vi "Vision Processing.vi"(4 "error in (no error)":errorcluster, 7 "Image Size Gear":T6=enum."160x120") -> ()   [LabVIEW 2016]
doc: "This VI runs in parallel to other tasks. It gets images from the camera, processes them for color or shape and use that information to affect robot behavior."
uses:
  Vision Support VIs/Camera Types.ctl
  <vilib>/Rock Robotics/WPI/Camera/WPI_CameraImageSize.ctl
  <vilib>/vision/Measure.llb/Edge Options.ctl
  <vilib>/vision/Measure.llb/Edge Polarity.ctl
  <vilib>/Rock Robotics/WPI/Camera/WPI_CameraWhite Balance Values.ctl
  <vilib>/Rock Robotics/WPI/Camera/WPI_CameraExposure Values.ctl
  <vilib>/Rock Robotics/WPI/Camera/WPI_CameraFrameRate.ctl
  <vilib>/Platform/TimedLoop/XDataNode/timing_clust.ctl
  <vilib>/Platform/TimedLoop/XDataNode/nitl_modes.ctl
  <vilib>/Platform/TimedLoop/XDataNode/wakeup.ctl
  <userlib>/836-libraries/Drive/Drive_Code/Drive_Code_Support/Sensor_Cluster.ctl
  <userlib>/836-libraries/Drive/Drive_Code/Drive_Code_Support/Camera_Cluster.ctl
  <userlib>/836-libraries/Drive/Drive_Code/Drive_Code_Support/Drive_Code_Notifier.ctl
  <userlib>/836-libraries/Drive/Drive_Code/Drive_Code_Support/Drive_Code_Command.ctl
  <userlib>/836-libraries/Drive/Drive_Code/Logging_Data.ctl
  <userlib>/836-libraries/Drive/Drive_Code/Drive_Code_Support/Drive_Code_PID_Bundle.ctl
  <vilib>/Rock Robotics/Network Tables/NT Write Boolean.vi
  <vilib>/platform/TimedLoop/XDataNode/XDataNode.xnode
  <vilib>/vision/NI_Vision_Development_Module.lvlib
  <vilib>/Platform/TimedLoop/XDataNode/XDNodeRunTimeDep.lvlib
panel:
  out "Mode 2":bool
  out "OOR 2":bool=TRUE
  out "GEAR cam":T1(graph)={"Distance (lateral)"=181.92766755741692, "Filtered"=0.0}
  in  "Rate Thresh 2":dbl=30.0 step=0.001
  in  "hi limit 2":dbl=100.0
  out "Distance (CT)":dbl=181.92766755741692
  in  "GearValid":dbl=40.0 format="%#_13g"
  in  "Gear Align % Y":dbl=70.0
  in  "Gear Align Offset (in)":dbl=30.0
  in  "Gear Tgt Sep":dbl=8.0
  in  "Gear Camera Orientation":cluster{"Yaw":dbl, "Elevation":dbl}={"Yaw"=0.0, "Elevation"=-2.0}
  out "Distance (lateral) 2":dbl=237.25608944267697
  out "Distance (lateral) 1":dbl=147.49292175195765
  in  "Hyster":dbl=0.3
  out "Mode":bool=TRUE
  out "OOR":bool
  in  "Rate Thresh":dbl=20.0 step=0.001
  in  "hi limit":dbl=50.0
  out "Waveform Chart":T2(graph)={"Distance (ft)"=inf, "Distance (ft)"=10.013263699521787, "Filtered"=10.013263699521787, "Double"=10.013263699521787}
  in  "Angle 2":enum16{"Horizontal", "Vertical", "Diagonal"}(ring)=enum."Vertical"
  out "Gear Yaw Delta":dbl=-2.9065025252525256
  in  "Boiler boresight":dbl=1.4
  in  "Edge Options Gear":T3={"Edge Polarity"=0, "Kernel Size"=3, "Width"=3, "Minimum Edge Strength"=15.0, "Interpolation Type"=enum."Bilinear Fixed", "Data Processing Method"=enum."Average"} {"Edge Polarity" items=["All Edges", "Rising Edges", "Falling Edges"]; "Minimum Edge Strength" format="%.2f"; "Width" step=2; "Kernel Size" step=2}
  in  "Gear boresight":dbl=-0.8
  in  "Ball?":bool=TRUE
  in  "LED Color Ball":T5={"Hue"={177.87863998678503, 241.41851407789423}, "Sat"={54.64285714285715, 255.0}, "Val"={37.39285714285715, 233.75}} {"Hue" scale=0.0..255.0 scale format="%#_3g"}
  in  "Brightness":i32=30
  in  "Exposure (%)":dbl format="%#_13g"
  in  "Color Temp (K)":dbl=4000.0 format="%#_13g"
  in  "Edge Options":T3={"Edge Polarity"=0, "Kernel Size"=3, "Width"=3, "Minimum Edge Strength"=20.0, "Interpolation Type"=enum."Bilinear Fixed", "Data Processing Method"=enum."Average"} {"Edge Polarity" items=["All Edges", "Rising Edges", "Falling Edges"]; "Minimum Edge Strength" format="%.2f"; "Width" step=2; "Kernel Size" step=2}
  in  "Size Limit %":dbl=0.04 format="%#_13g"
  in  "Cal Turret":bool
  out "Calibration error 2":errorcluster={"status"=TRUE, "code"=-1074396074, "source"=""}
  out "Physical Paths":string[](array[string])=["-0_1_1_1_0", "-0_1_2_1_0"]
  out "Logical Paths":string[](array[string])=["video0", "video1"]
  out "Gear Valid":bool
  out "Boiler Yaw Delta":dbl=-28.4328125
  out "Boiler Valid":bool
  out "Boiler Distance":dbl=inf
  in  "Angle":enum16{"Horizontal", "Vertical", "Diagonal"}(ring)=enum."Vertical"
  in  "Gear?":bool
  in  "Image SizeTurr":T6=enum."160x120"
  in  "Score Cutoff Turret":dbl=70.0
  in  "FOV":cluster{"X (degrees)":dbl, "Y (degrees)":dbl}={"X (degrees)"=61.0, "Y (degrees)"=34.3}
  in  "Height":T7={"Hc (GND to lense)"=4.25, "Ht (GND to CTR)"=13.25}
  in  "LED Color Target":T5={"Hue"={161.40152626725316, 238.59547054989036}, "Sat"={51.60714285714287, 255.0}, "Val"={18.071428571428584, 255.0}} {"Hue" scale=0.0..255.0 scale format="%#_3g"}
  in  "Camera Type":T8=enum."1013"
  in  "Score Cutoff %":dbl=50.0
  in  "Particles":dbl=5.0
  in  "Color Mode":u16(ring)=3 items=["RGB", "HSL", "HSV", "HSI"]
  in  "Use Calibration":bool
  out "Calibration error":errorcluster
  in  "Line Border":cluster{"Top":dbl, "Bottom":dbl}={"Top"=6.0, "Bottom"=1.0}
  in  "Display Original":bool=TRUE
  in  "Display Mask":bool=TRUE
  out "Mask":T9(plugin-control)
  out "Original Image":T9(plugin-control)
  out "loop ms":u32=100
  # "GEAR"
  # "TURRET"
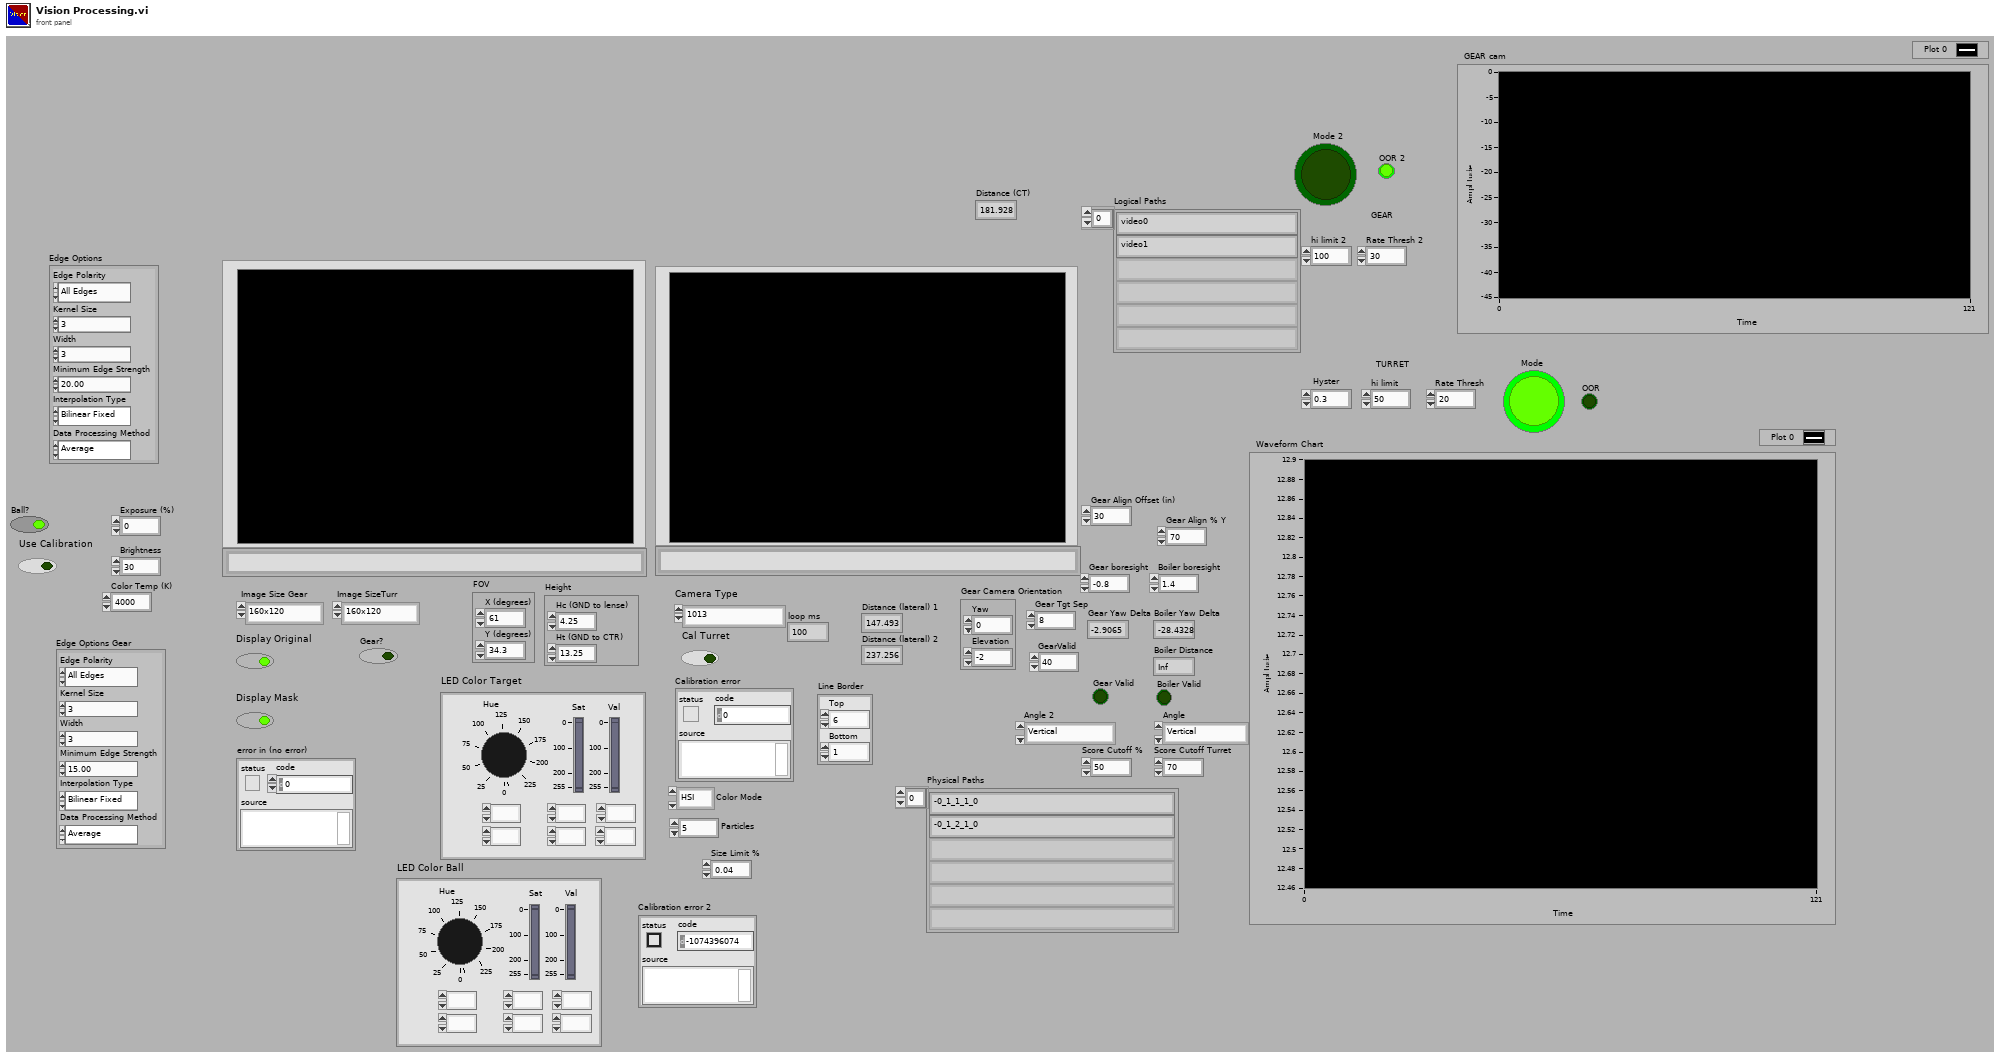
[diagram p1: front panel]
types:
  T1 = cluster{"Distance (lateral)":dbl, "Filtered":dbl}
  T2 = cluster{"Distance (ft)":dbl, "Distance (ft)":dbl, "Filtered":dbl, "Double":dbl}
  T3 = typedef "Edge Options.ctl" = cluster{"Edge Polarity":T4, "Kernel Size":u32, "Width":u32, "Minimum Edge Strength":sgl, "Interpolation Type":enum32{"Zero Order", "Bilinear", "Quadratic", "Cubic", "Bilinear Fixed"}, "Data Processing Method":enum32{"Average", "Median"}}
  T4 = typedef "Edge Polarity.ctl" = u32
  T5 = cluster{"Hue":cluster{dbl, dbl}, "Sat":cluster{dbl, dbl}, "Val":cluster{dbl, dbl}}
  T6 = typedef "WPI_CameraImageSize.ctl" = enum16{"640x480", "320x240", "160x120", "Custom"}
  T7 = cluster{"Hc (GND to lense)":dbl, "Ht (GND to CTR)":dbl}
  T8 = typedef "Camera Types.ctl" = enum16{"206", "1011", "1013", "MS HD3000 square", "MS HD3000 640x480"}
  T9 = typedef "IMAQ Image.ctl" = refnum<image>
  T10 = typedef "Image Type" = u32
  T11 = typedef "WPI_CameraFrameRate.ctl" = u32
  T12 = typedef "WPI_CameraExposure Values.ctl" = enum16{"Auto", "Flicker-free 50 Hz", "Flicker-free 60 Hz", "Hold current", "Custom"}
  T13 = typedef "WPI_CameraWhite Balance Values.ctl" = enum16{"Auto", "Fixed indoor", "Fixed outdoor 1", "Fixed outdoor 2", "Fixed fluorescent 1", "Fixed fluorescent 2", "Hold current", "Custom"}
  T14 = typedef "Particle Parameters" = i32
  T15 = typedef "WPI_CameraDevRef.ctl" = cluster{"Camera Address":string, "CameraStatus":errorcluster}
  T16 = typedef "XDNodeRunTimeDep.lvlib/timing_clust.ctl" = cluster{"Expected End [f-1]":u64, "Actual End [f-1]":u64, "Finished Late? [f-1]":bool, "Expected End [i-1]":u64, "Actual End [i-1]":u64, "Finished Late? [i-1]":bool, "Expected Start [i]":u64, "Actual Start [i]":u64, "Expected Start [f]":u64, "Actual Start [f]":u64, "Source Name":string, "Structure Name":string, "Period":i64, "Deadline":i64, "Offset":i64, "Start":i64, "Priority":i32, "Timeout":i32, "Mode":T17, "Wakeup Reason":T18, "Error":errorcluster, "Source Type":string, "Secondary Source Type":string, "Global End Time":u64, "Global Start Time":u64, "Frame Duration":u64, "Iteration Duration":u64, "Assigned CPU":i32, "I/O Scan Engine Mode":u32}
  T17 = typedef "XDNodeRunTimeDep.lvlib/nitl_modes.ctl" = enum32{"No Change", "Process missed periods, maintain original phase", "Discard missed periods, maintain original phase", "Process missed periods, ignore original phase", "Discard missed periods, ignore original phase"}
  T18 = typedef "XDNodeRunTimeDep.lvlib/wakeup.ctl" = enum32{"Normal", "Aborted", "Asynchronous wakeup", "Timing source error", "Timed loop error", "Timeout"}
  T19 = typedef "Sensor_Cluster.ctl" = cluster{"Gyro Data":cluster{"Gyro RT FIFO":refnum<k33>, "Gyro Current":dbl, "Gyro Hold":dbl}, "Encoder Data":cluster{"Encoder RT FIFO":refnum<k33>, "Encoder Current":dbl, "Encoder Hold":dbl}, "Camera Data":cluster{"Camera RT FIFO":refnum<k33>, "Camera Current":T20}}
  T20 = typedef "Camera_Cluster.ctl" = cluster{" Angle":dbl, "Valid":bool}
  T21 = cluster{"Cluster":T19, "Drive Command rt fifo":refnum<k33>, "Logging Data":refnum<k33>, "PID Update":refnum<notifier>}
  T22 = cluster{"Left":dbl, "Top":dbl, "Right":dbl, "Bottom":dbl}
  T23 = cluster{"Distance (ft)":dbl, "Score":dbl, "Normalized":cluster{"Center":cluster{dbl, dbl}, "Rectangle":cluster{"Numeric":dbl, "Numeric 2":dbl, "Numeric 3":dbl, "Numeric 5":dbl}}, "Pixels":cluster{"Center":cluster{dbl, dbl}, "Rectangle":cluster{"Numeric":dbl, "Numeric 2":dbl, "Numeric 3":dbl, "Numeric 5":dbl}}}
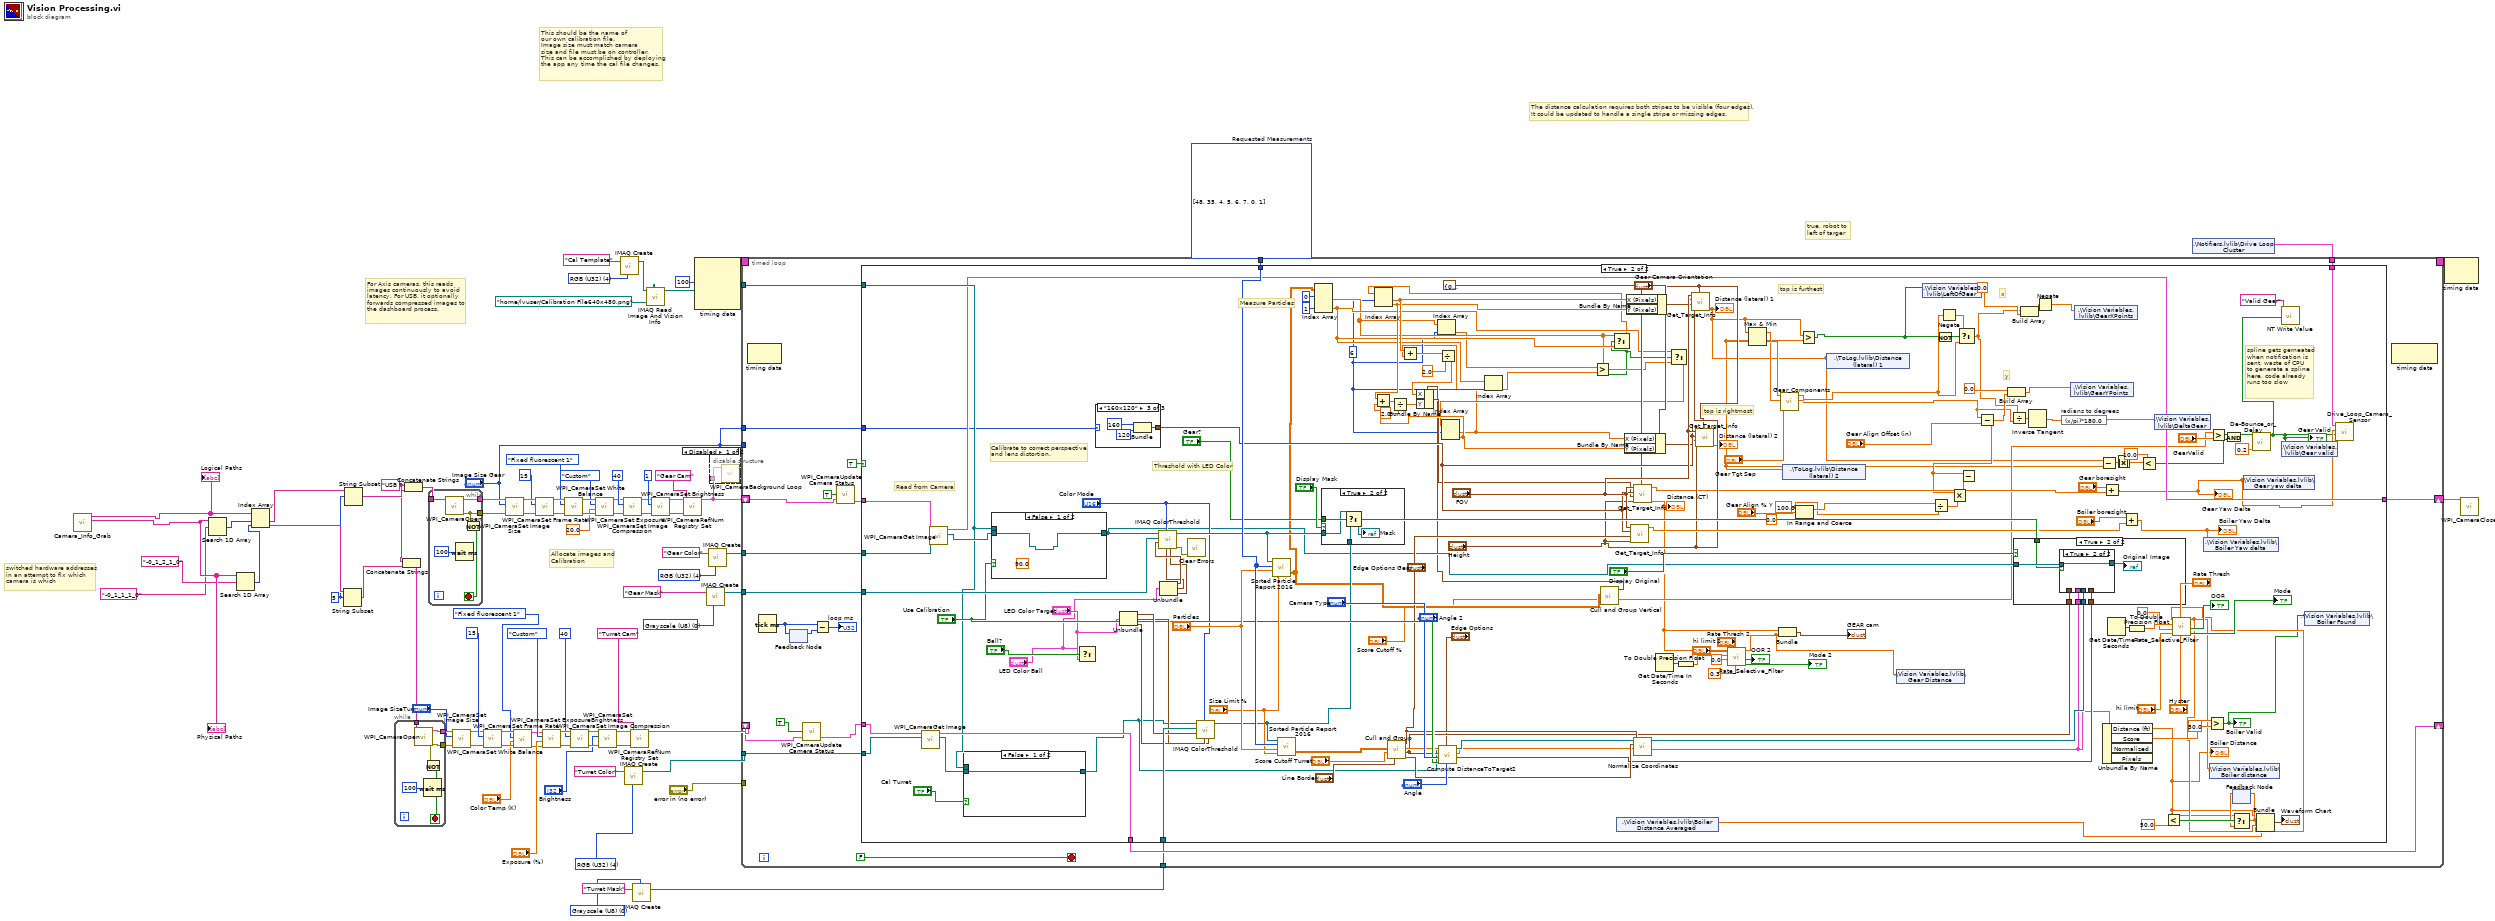
[diagram p0: block diagram]
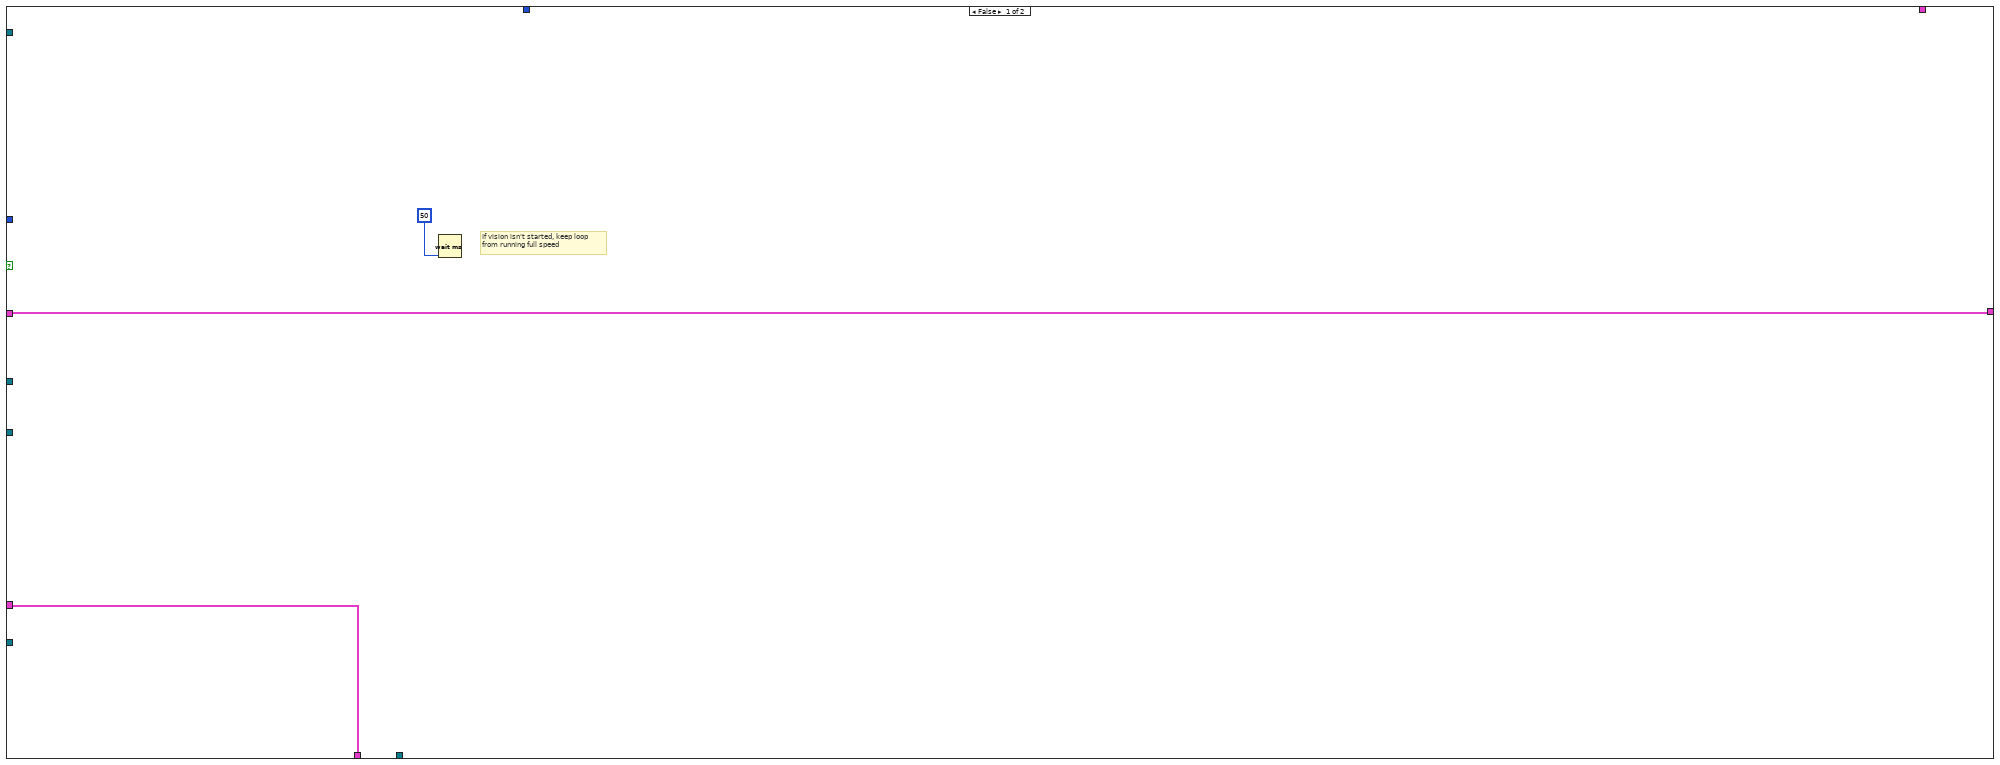
[diagram p2: hidden frame]
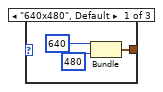
[diagram p3: hidden frame]
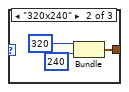
[diagram p4: hidden frame]
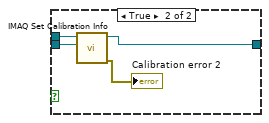
[diagram p5: hidden frame]
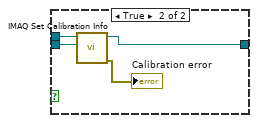
[diagram p9: hidden frame]
diagram:
  w19 = "USB " ("string")
  w21 = 5 ("offset (0)")
  w28 = T10 0 items=["Grayscale (U8)", "Grayscale (I16)", "Grayscale (SGL)", "Complex (CSG)", "RGB (U32)", "HSL (U32)", "RGB (U64)", "Grayscale (U16)"] ("Image Type")
  w30 = T10 4 items=["Grayscale (U8)", "Grayscale (I16)", "Grayscale (SGL)", "Complex (CSG)", "RGB (U32)", "HSL (U32)", "RGB (U64)", "Grayscale (U16)"] ("Image Type")
  w76 = T10 4 items=["Grayscale (U8)", "Grayscale (I16)", "Grayscale (SGL)", "Complex (CSG)", "RGB (U32)", "HSL (U32)", "RGB (U64)", "Grayscale (U16)"] ("Image Type")
  w81 = T10 0 items=["Grayscale (U8)", "Grayscale (I16)", "Grayscale (SGL)", "Complex (CSG)", "RGB (U32)", "HSL (U32)", "RGB (U64)", "Grayscale (U16)"] ("Image Type")
  w82 = T10 4 items=["Grayscale (U8)", "Grayscale (I16)", "Grayscale (SGL)", "Complex (CSG)", "RGB (U32)", "HSL (U32)", "RGB (U64)", "Grayscale (U16)"] ("Image Type")
  w78 = T14[] [48, 35, 4, 5, 6, 7, 0, 1] items=["Center of Mass X", "Center of Mass Y", "First Pixel X", "First Pixel Y", "Bounding Rect Left", "Bounding Rect Top", "Bounding Rect Right", "Bounding Rect Bottom", "Max Feret Diameter Start X", "Max Feret Diameter Start Y", "Max Feret Diameter End X", "Max Feret Diameter End Y", "Max Horiz. Segment Length Left", "Max Horiz. Segment Length Right", "Max Horiz. Segment Length Row", "-", "Bounding Rect Width", "Bounding Rect Height", "Bounding Rect Diagonal", "Perimeter", "Convex Hull Perimeter", "Holes' Perimeter", "Max Feret Diameter", "Equivalent Ellipse Major Axis", "Equivalent Ellipse Minor Axis", "Equivalent Ellipse Minor Axis (Feret)", "Equivalent Rect Long Side", "Equivalent Rect Short Side", "Equivalent Rect Diagonal", "Equivalent Rect Short Side (Feret)", "Average Horiz. Segment Length", "Average Vert. Segment Length", "Hydraulic Radius", "Waddel Disk Diameter", "-", "Area", "Holes' Area", "Particle & Holes' Area", "Convex Hull Area", "Image Area", "-", "Number of Holes", "Number of Horiz. Segments", "Number of Vert. Segments", "-", "Orientation", "Max Feret Diameter Orientation", "-", "% Area/Image Area", "% Area/(Particle & Holes' Area)", "Ratio of Equivalent Ellipse Axes", "Ratio of Equivalent Rect Sides", "-", "Elongation Factor", "Compactness Factor", "Heywood Circularity Factor", "Type Factor", "-", "Sum X", "Sum Y", "Sum XX", "Sum XY", "Sum YY", "Sum XXX", "Sum XXY", "Sum XYY", "Sum YYY", "-", "Moment of Inertia XX", "Moment of Inertia XY", "Moment of Inertia YY", "Moment of Inertia XXX", "Moment of Inertia XXY", "Moment of Inertia XYY", "Moment of Inertia YYY", "Norm. Moment of Inertia XX", "Norm. Moment of Inertia XY", "Norm. Moment of Inertia YY", "Norm. Moment of Inertia XXX", "Norm. Moment of Inertia XXY", "Norm. Moment of Inertia XYY", "Norm. Moment of Inertia YYY", "Hu Moment 1", "Hu Moment 2", "Hu Moment 3", "Hu Moment 4", "Hu Moment 5", "Hu Moment 6", "Hu Moment 7"]  # Requested Measurements
  # "true, robot to \nleft of targer"
  # "switched hardware addresses\nin an attempt to flx which\ncamera is which"
  # "For Axis cameras, this reads\nimages continuously to avoid\nlatency. For USB, it optionally\nforwards compressed images to\nthe dashboard process."
  # "Allocate images and\nCalibration"
  # "The distance calculation requires both stripes to be visible (four edges).\nIt could be updated to handle a single stripe or missing edges."
  # "This should be the name of \nour own calibration file.\nImage size must match camera\nsize and file must be on controller.\nThis can be accomplished by deploying\nthe app any time the cal file changes."
  n1 = call <userlib>:"Camera_Info_Grab.vi"() -> ("Physical Paths"=w14:string[], "Logical Paths"=w15:string[])  [unwired: 10 in]
  "Logical Paths" <- w15
  "Physical Paths" <- w14
  n2 = Search 1D Array(1D array=w14, element="-0_1_1_1_0") -> (index of element=w25:i32)  [unwired: 1 in]
  n3 = Search 1D Array(1D array=w14, element="-0_1_2_1_0") -> (index of element=w24:i32)  [unwired: 1 in]
  n4 = Index Array(array=w15, index #1=w25, index #2=w24) -> (element #1=w23:string, element #2=w22:string)
  n5 = String Subset(string=w22, offset (0)=w21) -> (substring=w18:string)  [unwired: 1 in]
  n6 = String Subset(string=w23, offset (0)=w21) -> (substring=w20:string)  [unwired: 1 in]
  n7 = Concatenate Strings(w19, w18) -> (w17:string)
  n8 = while {
    tunnel: [w87] -> w41
    tunnel: [w90] -> w40
    tunnel: w17 -> [w89]
    stop <- w86 stop-if-true
    n9 = call <vilib>:"WPI_CameraOpen.vi"("Camera Address"=w89) -> ("error out"=w87:errorcluster, "CameraDevRef"=w90:T15)  [unwired: 1 in, 8 out]
    n10 = Not(x=w87) -> (.not. x?=w86:bool)
    n11 = Wait (ms)(milliseconds to wait=u32 100) -> ()  [unwired: 1 out]
  }
  n12 = Concatenate Strings(w19, w20) -> (w16:string)
  n13 = while {
    tunnel: [w95] -> w63
    tunnel: [w92] -> w62
    tunnel: w16 -> [w94]
    stop <- w91 stop-if-true
    n14 = call <vilib>:"WPI_CameraOpen.vi"("Camera Address"=w94) -> ("error out"=w92:errorcluster, "CameraDevRef"=w95:T15)  [unwired: 1 in, 8 out]
    n15 = Wait (ms)(milliseconds to wait=u32 100) -> ()  [unwired: 1 out]
    n16 = Not(x=w92) -> (.not. x?=w91:bool)
  }
  n17 = call <vilib>:"WPI_CameraSet Image Size.vi"("error in (no error)"=w41, "Image Size"="Image SizeTurr", "CameraDevRef"=w40) -> ("error out"=w42:errorcluster, "CameraDevRef Out"=w39:T15)  [unwired: 1 in, 6 out]
  n18 = call <vilib>:"WPI_CameraSet Frame Rate.vi"("error in (no error)"=w42, "Frame Rate (fps)"=T11 15, "CameraDevRef"=w39) -> ("error out"=w10:errorcluster, "CameraDevRef Out"=w12:T15)  [unwired: 7 out]
  n19 = call <vilib>:"WPI_CameraSet Image Size.vi"("error in (no error)"=w62, "Image Size"="Image Size Gear", "CameraDevRef"=w63) -> ("error out"=w61:errorcluster, "CameraDevRef Out"=w64:T15)  [unwired: 1 in, 6 out]
  n20 = call <vilib>:"WPI_CameraSet White Balance.vi"("error in (no error)"=w10, "Color Temp (K)"="Color Temp (K)", "White Balance"=WPI_CameraWhite_Balance_Values."Fixed fluorescent 1", "CameraDevRef"=w12) -> ("error out"=w9:errorcluster, "CameraDevRef Out"=w11:T15)  [unwired: 6 in]
  n21 = call <vilib>:"WPI_CameraSet Frame Rate.vi"("error in (no error)"=w61, "Frame Rate (fps)"=T11 15, "CameraDevRef"=w64) -> ("error out"=w60:errorcluster, "CameraDevRef Out"=w66:T15)  [unwired: 7 out]
  n22 = call <vilib>:"WPI_CameraSet Exposure.vi"("error in (no error)"=w9, "Exposure (%)"="Exposure (%)", "Exposure"=WPI_CameraExposure_Values."Custom", "CameraDevRef"=w11) -> ("error out"=w43:errorcluster, "CameraDevRef Out"=w37:T15)  [unwired: 6 out]
  n23 = call <vilib>:"WPI_CameraSet White Balance.vi"("error in (no error)"=w60, "White Balance"=WPI_CameraWhite_Balance_Values."Fixed fluorescent 1", "CameraDevRef"=w66) -> ("error out"=w59:errorcluster, "CameraDevRef Out"=w65:T15)  [unwired: 1 in, 6 out]
  n24 = call <vilib>:"WPI_CameraSet Image Compression.vi"("error in (no error)"=w43, "Compression"=40, "CameraDevRef"=w37) -> ("error out"=w44:errorcluster, "CameraDevRef Out"=w38:T15)  [unwired: 7 out]
  n25 = call <vilib>:"WPI_CameraSet Exposure.vi"("error in (no error)"=w59, "Exposure (%)"=20.0, "Exposure"=WPI_CameraExposure_Values."Custom", "CameraDevRef"=w65) -> ("error out"=w58:errorcluster, "CameraDevRef Out"=w68:T15)  [unwired: 6 out]
  n26 = call <vilib>:"WPI_CameraSet Brightness.vi"("error in (no error)"=w44, "Brightness"="Brightness", "CameraDevRef"=w38) -> ("error out"=w45:errorcluster, "CameraDevRef Out"=w32:T15)  [unwired: 7 out]
  n27 = call "IMAQ Create"("Image Name"="Cal Template", "Image Type"=w76) -> ("New Image"=w74:T9)  [unwired: 2 in, 2 out]
  n28 = call <vilib>:"WPI_CameraSet Image Compression.vi"("error in (no error)"=w58, "Compression"=40, "CameraDevRef"=w68) -> ("error out"=w57:errorcluster, "CameraDevRef Out"=w67:T15)  [unwired: 7 out]
  n29 = call "IMAQ Create"("Image Name"="Turret Color", "Image Type"=w30) -> ("New Image"=w29:T9)  [unwired: 2 in, 2 out]
  n30 = call <vilib>:"WPI_CameraRefNum Registry Set.vi"("error in (no error)"=w45, "refnum name"="Turret Cam", "CameraDevRef"=w32) -> ("CameraDevRef"=w3:T15)  [unwired: 1 in, 7 out]
  n31 = call "IMAQ Create"("Image Name"="Turret Mask", "Image Type"=w28) -> ("New Image"=w26:T9)  [unwired: 2 in, 2 out]
  n32 = call "IMAQ Read Image And Vision Info"("File Path"=path "/home/lvuser/Calibration File640x480.png" ("Folder Location"), "Image"=w74) -> ("Image Out"=w73:T9)  [unwired: 7 in, 2 out]
  n33 = call <vilib>:"WPI_CameraSet Brightness.vi"("error in (no error)"=w57, "Brightness"=1, "CameraDevRef"=w67) -> ("error out"=w56:errorcluster, "CameraDevRef Out"=w72:T15)  [unwired: 7 out]
  n34 = call <vilib>:"WPI_CameraRefNum Registry Set.vi"("error in (no error)"=w56, "refnum name"="Gear Cam", "CameraDevRef"=w72) -> ("CameraDevRef"=w52:T15)  [unwired: 1 in, 7 out]
  n35 = node-c288(i64 100 ("Period")) -> (w85:T16)  [unwired: 3 in]
  n36 = call "IMAQ Create"("Image Name"="Gear Mask", "Image Type"=w81) -> ("New Image"=w79:T9)  [unwired: 2 in, 2 out]
  n37 = call "IMAQ Create"("Image Name"="Gear Color", "Image Type"=w82) -> ("New Image"=w77:T9)  [unwired: 2 in, 2 out]
  n38 = disable-structure shown="Disabled" {
    disable-tunnel: w52 -> [w96 _]
    frame Disabled {
      n39 = call <vilib>:"WPI_CameraBackground Loop.vi"("CameraDevRef"=w96) -> ()  [unwired: 11 in]
    }
    frame Enabled {
    }
  }
  n40 = shared-variable ".\\Notifiers.lvlib\\Drive Loop Cluster"() -> (w4:T21)  [unwired: 1 in, 1 out]
  n41 = timed-loop {
    tunnel: w77 -> [w113]
    tunnel: w79 -> [w116]
    tunnel: w78 -> [w115]
    tunnel: w73 -> [w114]
    shift-right: [w112] -> w51
    shift-left: w52 -> [w111]
    tunnel: "error in (no error)" -> [_]
    tunnel: "Image Size Gear" -> [_]
    shift-right: [w106] -> _
    shift-left: w3 -> [w101]
    tunnel: w29 -> [w105]
    tunnel: w26 -> [w104]
    timing: w85 -> [_]
    timing-out: [_] -> w84
    tunnel: "Image Size Gear" -> [w98]
    tunnel: w4 -> [w97]
    stop <- FALSE ("Boolean") stop-if-true
    n42 = node-c288() -> ()  [unwired: 1 in, 1 out]
    n43 = Tick Count (ms)() -> (millisecond timer value=w108:u32)
    n44 = feedback-in #1(w108) -> ()
    n45 = feedback #1() -> (w109:u32)  [unwired: 1 in]
    n46 = call <vilib>:"WPI_CameraUpdate Camera Status.vi"("CameraDevRef In"=w101, "Enable Vision"=TRUE) -> ("CameraDevRef Out"=w99:T15)  [unwired: 3 in]
    n47 = Subtract(x=w108, y=w109) -> (x-y=→"loop ms":u32)
    n48 = call <vilib>:"WPI_CameraUpdate Camera Status.vi"("CameraDevRef In"=w111, "Enable Vision"=TRUE) -> ("CameraDevRef Out"=w110:T15)  [unwired: 3 in]
    n49 = case shown="True" TRUE {
      tunnel: w116 -> [_ w278]
      tunnel: w115 -> [_ w268]
      tunnel: w114 -> [_ w240]
      tunnel: w110 -> [w122 w277]
      tunnel: w113 -> [_ w273]
      tunnel: [w122 w235] -> w112
      tunnel: w99 -> [w120 w276]
      tunnel: [w120 w275] -> w106
      tunnel: w105 -> [_ w274]
      tunnel: w104 -> [_ w272]
      tunnel: w98 -> [_ w214]
      tunnel: w97 -> [_ w175]
      frame False {
        # "If vision isn't started, keep loop\nfrom running full speed"
        n50 = Wait (ms)(milliseconds to wait=u32 50) -> ()  [unwired: 1 out]
      }
      frame True {
        w194 = 100.0 ("upper limit")
        w211 = cluster{"X (Pixels)":dbl, "Y (Pixels)":dbl} {"X (Pixels)"=0.0, "Y (Pixels)"=0.0} ("Target Location")
        w137 = 6 ("index")
        # "spline gets gerneated\nwhen notification is\nsent, waste of CPU\nto generate a spline\nhere, code already\nruns too slow"
        # "y"
        # "x"
        # "top is furthest"
        # "top is rightmost"
        # "Read from Camera"
        # "Calibrate to correct perspective\nand lens distortion."
        # "Measure Particles"
        # "Threshold with LED Color"
        n51 = call <vilib>:"WPI_CameraGet Image.vi"("Image"=w274, "CameraDevRef"=w276) -> ("Image Out"=w239:T9, "CameraDevRef Out"=w275:T15)  [unwired: 7 in, 1 out]
        n52 = call <vilib>:"WPI_CameraGet Image.vi"("Image"=w273, "CameraDevRef"=w277) -> ("Image Out"=w249:T9, "CameraDevRef Out"=w235:T15)  [unwired: 7 in, 1 out]
        n53 = case shown="False" "Cal Turret" {
          tunnel: [w288 w292] -> w238
          tunnel: w239 -> [w288 w291]
          tunnel: w240 -> [_ w290]
          frame False {
          }
          frame True {
            n54 = call "IMAQ Set Calibration Info"("Image Dst"=w291, "Image Src"=w290) -> ("error out"=→"Calibration error 2":errorcluster, "Calibrated Image"=w292:T9)  [unwired: 8 in]
          }
        }
        n55 = case shown="False" "Use Calibration" {
          tunnel: [w306 w310] -> w156
          tunnel: w249 -> [w306 w309]
          tunnel: w240 -> [_ w308]
          frame False {
            (unwired) sgl 90.0 ("Angle (degrees)")
          }
          frame True {
            n56 = call "IMAQ Set Calibration Info"("Image Dst"=w309, "Image Src"=w308) -> ("error out"=→"Calibration error":errorcluster, "Calibrated Image"=w310:T9)  [unwired: 8 in]
          }
        }
        n57 = Select(t="LED Color Ball", s="Ball?", f="LED Color Target") -> ()  [unwired: 1 out]
        n58 = case shown="\"160x120\"" w214 {
          tunnel: [w279 w282 w285] -> w209
          frame "640x480", Default {
            n59 = Bundle(640, 480) -> (w279:cluster{i32, i32})  [unwired: 1 in]
          }
          frame "320x240" {
            n60 = Bundle(320, 240) -> (w282:cluster{i32, i32})  [unwired: 1 in]
          }
          frame "160x120" {
            n61 = Bundle(160, 120) -> (w285:cluster{i32, i32})  [unwired: 1 in]
          }
        }
        n62 = Unbundle("LED Color Target") -> ("Hue"=w271:cluster{dbl, dbl}, "Sat"=w270:cluster{dbl, dbl}, "Val"=w269:cluster{dbl, dbl})
        n63 = Unbundle("LED Color Ball") -> ("Hue"=w168:cluster{dbl, dbl}, "Sat"=w167:cluster{dbl, dbl}, "Val"=w166:cluster{dbl, dbl})
        n64 = call "IMAQ ColorThreshold"("Blue or Luma or Val or Inten Range"=w166, "Green or Sat Range"=w167, "Color Mode"="Color Mode", "Red or Hue Range"=w168, "Image Dst"=w278, "Image Src"=w156) -> ("error out"=w253:errorcluster, "Image Dst Out"=w252:T9)  [unwired: 4 in]
        n65 = call <vilib>:"Clear Errors.vi"("error in (no error)"=w253) -> ()  [unwired: 5 in, 2 out]
        n66 = call "IMAQ ColorThreshold"("Blue or Luma or Val or Inten Range"=w269, "Green or Sat Range"=w270, "Color Mode"="Color Mode", "Red or Hue Range"=w271, "Image Dst"=w272, "Image Src"=w238) -> ("Image Dst Out"=w246:T9)  [unwired: 4 in, 1 out]
        n67 = call "Sorted Particle Report 2016.vi"("Min Area Size %"="Size Limit %", "Particle Count Limit"="Particles", "Pixel Measurements"=w268, "Image in"=w252) -> ("Sorted Data"=w155:dbl[][])  [unwired: 1 out]
        n68 = call "Sorted Particle Report 2016.vi"("Min Area Size %"="Size Limit %", "Particle Count Limit"="Particles", "Pixel Measurements"=w268, "Image in"=w246) -> ("Sorted Data"=w261:dbl[][])  [unwired: 1 out]
        n69 = Index Array(array=w155, index (row) #1=0 ("index (row)"), index (row) #2=1 ("index (row)")) -> (element #1=w139:dbl[], element #2=w142:dbl[])  [unwired: 2 in]
        n70 = case shown="True" "Display Mask" {
          tunnel: w252 -> [_ w303]
          tunnel: "Gear?" -> [_ w305]
          tunnel: w246 -> [_ w302]
          frame False {
          }
          frame True {
            n71 = Select(t=w303, s=w305, f=w302) -> (s? t:f=→"Mask":T9)
          }
        }
        n72 = call "Cull and Group.vi"("Line Border"="Line Border", "Score Cutoff"="Score Cutoff Turret", "Sorted Data"=w261) -> ("Rect"=w258:T22, "Line"=w244:T22, "Score"=w257:dbl, "Center"=w245:cluster{"X":dbl, "Y":dbl})  [unwired: 5 in]
        n73 = Index Array(array=w139, index=w137) -> (element=w138:dbl)
        n74 = call "Compute DistanceToTarget2.vi"("Angle"="Angle", "Edge Options"="Edge Options", "Calibrated"="Use Calibration", "Camera Type"="Camera Type", "Line"=w244, "Image Src"=w238) -> ("Edges"=w243:cluster{"X":sgl, "Y":sgl}[], "Distance (ft)"=w256:dbl, "Image Dst Out"=w259:T9)  [unwired: 3 in]
        n75 = Index Array(array=w142, index=w137) -> (element=w141:dbl)
        n76 = Greater?(x=w138, y=w141) -> (0:w134:bool)
        n77 = call "Cull and Group Vertical.vi"("Score Cutoff"="Score Cutoff %", "Sorted Data"=w155) -> ("Top Score"=w153:dbl, "Center"=w154:cluster{"X":dbl, "Y":dbl})  [unwired: 6 in, 2 out]
        n78 = Select(t=w139, s=w134, f=w142) -> (s? t:f=w136:dbl[])
        n79 = Index Array(array=w136, index #1=w137) -> (element #1=w186:dbl, element #2=w182:dbl)  [unwired: 1 in]
        n80 = shared-variable ".\\Vision Variables.lvlib\\Boiler Distance Averaged"() -> (w215:dbl)  [unwired: 1 in, 1 out]
        n81 = Bundle By Name(cluster=w211, "X (Pixels)"=w186, "Y (Pixels)"=w182) -> (w207:cluster{"X (Pixels)":dbl, "Y (Pixels)":dbl})
        n82 = call "Get_Target_Info.vi"("Height"="Height", "Target Location"=w245, "Resolution"=w209, "FOV"="FOV") -> ("Yaw Delta"=w231:dbl)  [unwired: 2 in, 5 out]
        n83 = call "Normalize Coordinates.vi"("Score"=w257, "Center"=w245, "Distance"=w256, "Bounding box"=w258, "Image in"=w259) -> ("Results"=w229:T23, "Image out"=w242:T9)  [unwired: 5 in]
        n84 = Get Date/Time In Seconds() -> (seconds since 1Jan1904=w165:timestamp)
        n85 = Select(t=w142, s=w134, f=w139) -> (s? t:f=w140:dbl[])
        n86 = Index Array(array=w140, index #1=w137) -> (element #1=w132:dbl, element #2=w181:dbl)  [unwired: 1 in]
        n87 = Add(x=w182, y=w181) -> (x+y=w180:dbl)
        n88 = Divide(x=w180, y=2.0) -> (x/y=w178:dbl)
        n89 = Add(x=w186, y=w132) -> (x+y=w185:dbl)
        n90 = Divide(x=w185, y=2.0) -> (x/y=w183:dbl)
        n91 = Bundle By Name(cluster=w154, "X"=w183, "Y"=w178) -> (w177:cluster{"X":dbl, "Y":dbl})
        n92 = Bundle By Name(cluster=w211, "X (Pixels)"=w132, "Y (Pixels)"=w181) -> (w208:cluster{"X (Pixels)":dbl, "Y (Pixels)":dbl})
        n93 = call "Get_Target_Info.vi"("Camera Orientation"="Gear Camera Orientation", "Height"="Height", "Target Location"=w177, "Resolution"=w209, "FOV"="FOV") -> ("Distance (lateral)"=w150:dbl, "Yaw Delta"=w187:dbl)  [unwired: 1 in, 4 out]
        "Distance (CT)" <- w150
        n94 = To Double Precision Float(number=w165) -> (double precision float=w164:dbl)
        n95 = call "Get_Target_Info.vi"("Camera Orientation"="Gear Camera Orientation", "Height"="Height", "Target Location"=w207, "Resolution"=w209, "FOV"="FOV") -> ("Distance (lateral)"=w127:dbl)  [unwired: 1 in, 5 out]
        "Distance (lateral) 1" <- w127
        n96 = call "Get_Target_Info.vi"("Camera Orientation"="Gear Camera Orientation", "Height"="Height", "Target Location"=w208, "Resolution"=w209, "FOV"="FOV") -> ("Distance (lateral)"=w126:dbl)  [unwired: 1 in, 5 out]
        "Distance (lateral) 2" <- w126
        n97 = call <userlib>:"Rate_Selective_Filter.vi"("Hyster"=0.3, "Rate Thresh"="Rate Thresh 2", "hi limit"="hi limit 2", "lo limit"=0.0, "Time"=w164, "Distance"=w150) -> ("Mode"=→"Mode 2":bool, "OOR"=→"OOR 2":bool, "Filtered"=w133:dbl)  [unwired: 1 in]
        n98 = Max & Min(x=w127, y=w126) -> (max(x,y)=w202:dbl, min(x,y)=w203:dbl)
        n99 = Bundle("Distance (lateral)"=w150, "Filtered"=w133) -> (→"GEAR cam":T1)  [unwired: 1 in]
        n100 = call "Gear_Components.vi"("Target Seperation"="Gear Tgt Sep", "Far Target Distance"=w202, "Close Target Distance"=w203) -> ("X Component"=w147:dbl, "Y Component"=w144:dbl)  [unwired: 7 in]
        n101 = shared-variable ".\\ToLog.lvlib\\Distance (lateral) 2"(w126) -> ()  [unwired: 1 in, 1 out]
        n102 = In Range and Coerce(upper limit=w194, x="Gear Align % Y", lower limit=0.0) -> (coerced(x)=w195:dbl)  [unwired: 1 out]
        n103 = Greater?(x=w127, y=w126) -> (0:w135:bool)
        n104 = shared-variable ".\\ToLog.lvlib\\Distance (lateral) 1"(w127) -> ()  [unwired: 1 in, 1 out]
        n105 = shared-variable ".\\Vision Variables.lvlib\\Gear Distance"(w133) -> ()  [unwired: 1 in, 1 out]
        n106 = shared-variable ".\\Vision Variables.lvlib\\LeftOfGear"(w135) -> ()  [unwired: 1 in, 1 out]
        n107 = Divide(x=w195, y=w194) -> (x/y=w193:dbl)
        n108 = Not(x=w135) -> (.not. x?=w200:bool)
        n109 = Negate(x=w147) -> (-x=w199:dbl)
        n110 = Select(t=w199, s=w200, f=w147) -> (s? t:f=w143:dbl)
        n111 = Subtract(x=w144, y="Gear Align Offset (in)") -> (x-y=w145:dbl)
        n112 = Multiply(x=w145, y=w193) -> (x*y=w189:dbl)
        n113 = Subtract(x=w145, y=w189) -> ()  [unwired: 1 out]
        n114 = Build Array(0.0 ("element"), w145) -> (w149:dbl[])
        n115 = Divide(x=w143, y=w144) -> (x/y=w191:dbl)
        n116 = case shown="True" "Display Original" {
          tunnel: w156 -> [_ w298]
          tunnel: "Gear?" -> [_ w297]
          tunnel: w244 -> [_ w296]
          tunnel: w243 -> [_ w295]
          tunnel: w242 -> [_ w294]
          tunnel: w229 -> [_ w293]
          frame False {
          }
          frame True {
            n117 = case shown="True" w297 {
              tunnel: [w300 w301] -> w299
              tunnel: w298 -> [_ w301]
              tunnel: w296 -> [_ _]
              tunnel: w295 -> [_ _]
              tunnel: w294 -> [w300 _]
              tunnel: w293 -> [_ _]
              frame False {
              }
              frame True {
              }
            }
            "Original Image" <- w299
          }
        }
        n118 = Build Array(w143, 0.0 ("element")) -> (w192:dbl[])
        n119 = Inverse Tangent(1:w191) -> (0:w188:dbl)
        n120 = Negate(x=w192) -> (-x=w148:dbl[])
        n121 = expression code="(x/pi)*180.0" "radians to degrees"(w188) -> (w176:dbl)
        n122 = shared-variable ".\\Vision Variables.lvlib\\GearYPoints"(w149) -> ()  [unwired: 1 in, 1 out]
        n123 = shared-variable ".\\Vision Variables.lvlib\\GearXPoints"(w148) -> ()  [unwired: 1 in, 1 out]
        n124 = Subtract(x=w127, y=w126) -> (x-y=w130:dbl)
        n125 = Unbundle By Name(w229) -> ("Distance (ft)"=w204:dbl, "Score"=w255:dbl)  [unwired: 2 out]
        "Boiler Distance" <- w204
        n126 = Add(x="Gear boresight", y=w187) -> (x+y=w171:dbl)
        "Gear Yaw Delta" <- w171
        n127 = Get Date/Time In Seconds() -> (seconds since 1Jan1904=w228:timestamp)
        n128 = Absolute Value(x=w130) -> (abs(x)=w129:dbl)
        n129 = Add(x="Boiler boresight", y=w231) -> (x+y=w230:dbl)
        "Boiler Yaw Delta" <- w230
        n130 = To Double Precision Float(number=w228) -> (double precision float=w227:dbl)
        n131 = Less?(x=w129, y=10.0) -> (x < y?=w125:bool)
        n132 = shared-variable ".\\Vision Variables.lvlib\\DeltaGear"(w176) -> ()  [unwired: 1 in, 1 out]
        n133 = Less?(x=w204, y=50.0) -> (x < y?=w220:bool)
        n134 = shared-variable ".\\Vision Variables.lvlib\\Boiler Yaw delta"(w230) -> ()  [unwired: 1 in, 1 out]
        n135 = Greater?(x=w255, y=50.0) -> (0:w205:bool)
        "Boiler Valid" <- w205
        n136 = Greater?(x=w153, y="GearValid") -> (0:w174:bool)
        n137 = And(x=w174, y=w125) -> (x .and. y?=w131:bool)
        n138 = feedback #2() -> (w219:dbl)  [unwired: 1 in]
        n139 = Select(t=w204, s=w220, f=w219) -> (s? t:f=w216:dbl)
        n140 = call <userlib>:"Rate_Selective_Filter.vi"("Hyster"="Hyster", "Rate Thresh"="Rate Thresh", "hi limit"="hi limit", "lo limit"=0.0, "Time"=w227, "Distance"=w216) -> ("Mode"=→"Mode":bool, "OOR"=→"OOR":bool, "Filtered"=w218:dbl)  [unwired: 1 in]
        n141 = shared-variable ".\\Vision Variables.lvlib\\Boiler distance"(w218) -> ()  [unwired: 1 in, 1 out]
        n142 = feedback-in #2(w216) -> ()
        n143 = shared-variable ".\\Vision Variables.lvlib\\Gear yaw delta"(w171) -> ()  [unwired: 1 in, 1 out]
        n144 = call <userlib>:"De-Bounce_or_Delay.vi"("Eval Period (sec)"=0.2, "Signal Input"=w131) -> ("Stable"=w124:bool)  [unwired: 9 in]
        "Gear Valid" <- w124
        n145 = Bundle("Distance (ft)"=w204, "Distance (ft)"=w216, "Filtered"=w218, "Double"=w215) -> (→"Waveform Chart":T2)  [unwired: 1 in]
        n146 = call-poly <vilib>:"NT Write Value.vi"("Boolean"=w124, "Name"="Valid Gear") -> ()  [unwired: 9 in, 1 out]
        n147 = shared-variable ".\\Vision Variables.lvlib\\Gear valid"(w124) -> ()  [unwired: 1 in, 1 out]
        n148 = shared-variable ".\\Vision Variables.lvlib\\Boiler Found"(w205) -> ()  [unwired: 1 in, 1 out]
        n149 = call <userlib>:"Drive_Loop_Camera_Sensor.vi"("Stable?"=w124, "Camera Angle"=w171, "Drive Loop Cluster"=w175) -> ()  [unwired: 9 in]
      }
    }
    n150 = node-c288() -> ()  [unwired: 1 in, 1 out]
  }
  n151 = node-c288(w84) -> ()  [unwired: 1 out]
  n152 = call <vilib>:"WPI_CameraClose.vi"("CameraDevRef"=w51) -> ()  [unwired: 1 in, 10 out]
